vi "Anlagengrenzwerte pruefen - PC.vi"(9 "Wert":dbl, 10 "Anlagen-Parametername":T1) -> (0 "AbschMax":bool, 1 "AbschMin":bool, 2 "WarnMax":bool, 3 "WarnMin":bool, 5 "F.Br.":bool)   [LabVIEW 2020, in "Stoerungen.lvlib"]
uses:
  Stoerungen.lvlib
  Seiten/Anlagengrenzwerte/Anlagen-Parameternamen.ctl
  Seiten/Anlagengrenzwerte/FGV Anlagengrenzwerte Aktionen.ctl
  Seiten/Anlagengrenzwerte/Anlagengrenzwerte.lvlib
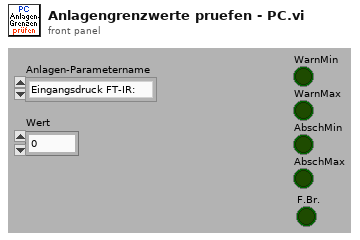
[diagram p1: front panel]
types:
  T1 = typedef "Anlagengrenzwerte.lvlib/Anlagen-Parameternamen.ctl" = enum16{"Eingangsdruck FT-IR:", "Durchfluss FT-IR:", "Durchfluss CalGas", "Druck Ausgang", "Druck Kalter Block", "Heizleitung intern", "Heizleitung zu FT-IR", "Heizung Filter:", "Heizung Pumpe:", "HL Extern SP1", "HL Extern SP2", "FT-IR Messzelle", "Schaltschrank", "Gaskühler"}
  T2 = typedef "Anlagengrenzwerte.lvlib/FGV Anlagengrenzwerte Aktionen.ctl" = enum16{"Lesen", "Grenzwerte schreiben"}
  T3 = typedef "Anlagengrenzwerte.lvlib/Anlagen-Grenzwerte Anzeige.ctl" = cluster{"Eingangsdruck FT-IR:":T4, "Durchfluss FT-IR:":T4, "Durchfluss CalGas:":T4, "Druck Ausgang:":T4, "Druck Kalter Block:":T4, "Heizleitungen intern:":T4, "Heizleitung zu FT-IR:":T4, "Heizung Filterblock:":T4, "Heizung Pumpe:":T4, "Heizleitung Extern SP1:":T4, "Heizleitung Extern SP2:":T4, "FT-IR Heizung Messzelle:":T4, "Schaltschranktemperatur:":T4, "Gaskühler:":T4}
  T4 = typedef "Anlagengrenzwerte.lvlib/Anlagen-Parameter Anzeige.ctl" = cluster{"Sollwert":sgl, "Warn-Min":sgl, "Warn-Max":sgl, "Abschalt-Min":sgl, "Abschalt-Max":sgl, "Regler":u16}
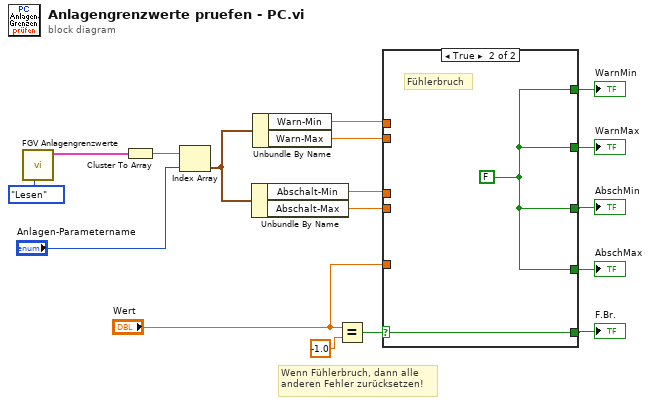
[diagram p0: block diagram]
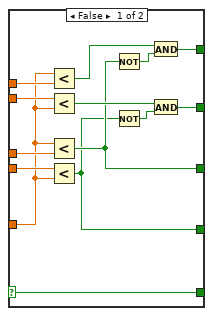
[diagram p2: hidden frame]
diagram:
  # "Wenn Fühlerbruch, dann alle \nanderen Fehler zurücksetzen!"
  n1 = call "FGV Anlagengrenzwerte.vi"("Aktion"=FGV_Anlagengrenzwerte_Aktionen."Lesen") -> ("Anlagen-Grenzwerte Anzeige"=w13:T3)  [unwired: 10 in]
  n2 = Cluster To Array(cluster=w13) -> (array=w17:T4[])
  n3 = Index Array(array=w17, index="Anlagen-Parametername") -> (element=w15:T4)
  n4 = Unbundle By Name(w15) -> ("Abschalt-Min"=w8:sgl, "Abschalt-Max"=w7:sgl)
  n5 = Unbundle By Name(w15) -> ("Warn-Min"=w10:sgl, "Warn-Max"=w9:sgl)
  n6 = Equal?(x="Wert", y=-1.0) -> (x = y?=w12:bool)
  n7 = case shown="True" w12 {
    selector: w12 -> [w18 w33]
    tunnel: w10 -> [w31 _]
    tunnel: w9 -> [w30 _]
    tunnel: w8 -> [w29 _]
    tunnel: w7 -> [w28 _]
    tunnel: [w23 w32] -> w1
    tunnel: [w22 w32] -> w2
    tunnel: [w21 w32] -> w3
    tunnel: [w20 w32] -> w4
    tunnel: "Wert" -> [w19 _]
    tunnel: [w18 w33] -> w5
    frame False {
      n8 = Less?(x=w19, y=w31) -> (x < y?=w27:bool)
      n9 = Less?(x=w30, y=w19) -> (x < y?=w24:bool)
      n10 = Less?(x=w19, y=w29) -> (x < y?=w21:bool)
      n11 = Less?(x=w28, y=w19) -> (x < y?=w20:bool)
      n12 = Not(x=w21) -> (.not. x?=w26:bool)
      n13 = Not(x=w20) -> (.not. x?=w25:bool)
      n14 = And(x=w27, y=w26) -> (x .and. y?=w23:bool)
      n15 = And(x=w24, y=w25) -> (x .and. y?=w22:bool)
    }
    frame True {
      w32 = FALSE
      # "Fühlerbruch"
    }
  }
  "WarnMin" <- w1
  "WarnMax" <- w2
  "AbschMin" <- w3
  "AbschMax" <- w4
  "F.Br." <- w5
